vi "Ultrasonic Loop.vi"   [LabVIEW 2014]
uses:
  Common Code/Ultrasonic Indicators.ctl
  <vilib>/Rock Robotics/WPI/Ultrasonic/WPI_UltrasonicRangeUnits.ctl
  Common Code/Change Detect Boolean.vi
  <vilib>/Rock Robotics/WPI/Ultrasonic/WPI_SonarSRF04DigitalRefNum Registry Get.vi
  <vilib>/Rock Robotics/WPI/Ultrasonic/WPI_SonarSRF04DigitalGetRange.vi
  <vilib>/addons/control/pid/pid.llb/PID Control Input Filter (DBL).vi
  Robot Global Data.vi
  <vilib>/addons/control/pid/NI_PID_pid.lvlib
types:
  T1 = typedef "WPI_UltrasonicRangeUnits.ctl" = enum16{"inches", "mm"}
  T2 = typedef "Ultrasonic Indicators.ctl" = cluster{"Left Distance":dbl, "Right Distance":dbl, "Center Distance":dbl, "Left Distance Unfilter":dbl, "Right Distance Unfilter":dbl, "Center Distance Unfilter":dbl}
  T3 = typedef "WPI_UltrasonicDeviceRef.ctl" = cluster{"DevStatus":errorcluster, "Ping Digital Controller":T4, "Echo Digital Controller":T4, "Ping Channel":T5, "Echo Channel":T5, "CntIndex":T6}
  T4 = typedef "FPGA_TypedefDigitalModule.ctl" = enum16{"Controller 1"}
  T5 = typedef "FPGA_DIOChannel.ctl" = enum8{"DIO 0", "DIO 1", "DIO 2", "DIO 3", "DIO 4", "DIO 5", "DIO 6", "DIO 7", "DIO 8", "DIO 9", "DIO MXP 0", "DIO MXP 1", "DIO MXP 2", "DIO MXP 3", "DIO MXP 4", "DIO MXP 5", "DIO MXP 6", "DIO MXP 7", "DIO MXP 8", "DIO MXP 9", "DIO MXP 10", "DIO MXP 11", "DIO MXP 12", "DIO MXP 13", "DIO MXP 14", "DIO MXP 15", "Invalid"}
  T6 = typedef "FPGA_CounterCtrSystemIndex.ctl" = enum8{"Ctr 0", "Ctr 1", "Ctr 2", "Ctr 3", "Ctr 4", "Ctr 5", "Ctr 6", "Ctr 7", "Invalid"}
  T7 = typedef "WPI_AnalogChannelDevRef.ctl" = cluster{"DevStatus":errorcluster, "Controller":T8, "Analog Channel":T9}
  T8 = typedef "FPGA_TypedefAnalogModule.ctl" = enum16{"Controller 1"}
  T9 = typedef "FPGA_AIChannel.ctl" = enum8{"AI 0", "AI 1", "AI 2", "AI 3", "AI MXP 0", "AI MXP 1", "AI MXP 2", "AI MXP 3", "Invalid"}
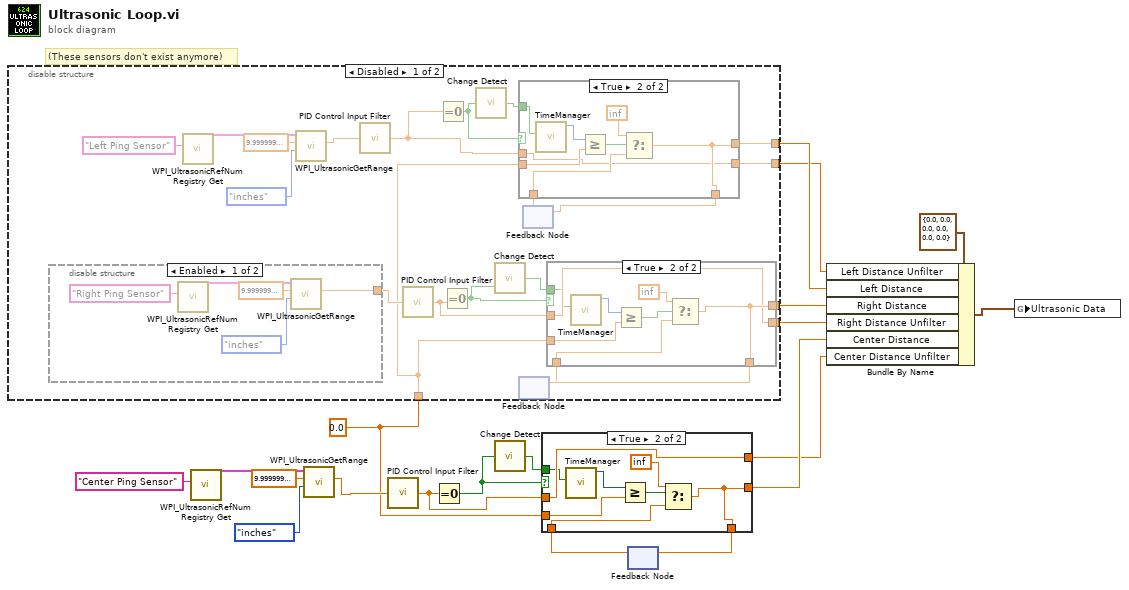
[diagram p0: block diagram]
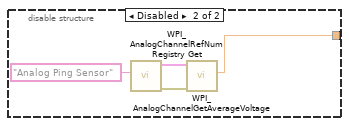
[diagram p4: hidden frame]
diagram:
  w1 = 0.0
  # "(These sensors don't exist anymore)"
  n1 = disable-structure shown="Disabled" {
    disable-tunnel: [w36 _] -> w17
    disable-tunnel: [w35 _] -> w16
    disable-tunnel: w1 -> [w26 _]
    disable-tunnel: [w25 _] -> w6
    disable-tunnel: [w24 _] -> w4
    frame Disabled {
      n2 = disable-structure shown="Enabled" {
        disable-tunnel: [w59 w64] -> w33
        frame Enabled {
          n3 = call-poly <vilib>:"WPI_UltrasonicRefNum Registry Get.vi"("refnum name"="Right Ping Sensor") -> ("SonarSRF04DevRef"=w62:T3)  [unwired: 9 in, 1 out]
          n4 = call-poly <vilib>:"WPI_UltrasonicGetRange.vi"("Range Units"=WPI_UltrasonicRangeUnits."inches", "ping time (s)"=sgl 1e-05, "SonarSRF04DevRef"=w62) -> ("Distance"=w59:dbl)  [unwired: 6 in, 2 out]
        }
        frame Disabled {
          n5 = call <vilib>:"WPI_AnalogChannelRefNum Registry Get.vi"("refnum name"="Analog Ping Sensor") -> ("error out"=w67:errorcluster, "AIDeviceRef"=w66:T7)  [unwired: 9 in]
          n6 = call <vilib>:"WPI_AnalogChannelGetAverageVoltage.vi"("error in (no error)"=w67, "AIDeviceRef"=w66) -> ("Voltage"=w64:dbl)  [unwired: 7 in, 2 out]
        }
      }
      n7 = call-poly <vilib>:"WPI_UltrasonicRefNum Registry Get.vi"("refnum name"="Left Ping Sensor") -> ("SonarSRF04DevRef"=w40:T3)  [unwired: 9 in, 1 out]
      n8 = call-poly <vilib>:"WPI_UltrasonicGetRange.vi"("Range Units"=WPI_UltrasonicRangeUnits."inches", "ping time (s)"=sgl 1e-05, "SonarSRF04DevRef"=w40) -> ("Distance"=w34:dbl)  [unwired: 6 in, 2 out]
      n9 = call-poly <vilib>:"PID Control Input Filter.vi"("input"=w34) -> ("output"=w31:dbl)  [unwired: 4 in]
      n10 = call-poly <vilib>:"PID Control Input Filter.vi"("input"=w33) -> ("output"=w32:dbl)  [unwired: 4 in]
      n11 = Equal To 0?(x=w31) -> (x = 0?=w23:bool)
      n12 = Equal To 0?(x=w32) -> (x = 0?=w21:bool)
      n13 = call-poly "Change Detect.vi"("In"=w23) -> ("Changed?"=w22:bool)
      n14 = call-poly "Change Detect.vi"("In"=w21) -> ("Changed?"=w20:bool)
      n15 = feedback #1() -> (w27:dbl)  [unwired: 1 in]
      n16 = feedback #2() -> (w29:dbl)  [unwired: 1 in]
      n17 = case shown="True" w23 {
        tunnel: [w41 w45] -> w35
        tunnel: w31 -> [w41 w43]
        tunnel: [w41 w45] -> w30
        tunnel: w29 -> [_ w46]
        tunnel: w26 -> [_ w44]
        tunnel: [w41 w43] -> w25
        tunnel: w22 -> [_ w42]
        frame False {
        }
        frame True {
          n18 = call "TimeManager.vi"("Reset?"=w42) -> ("Time Since Reset"=w49:u32)  [unwired: 9 in, 1 out]
          n19 = Greater Or Equal?(x=w49, y=w44) -> (x >= y?=w47:bool)
          n20 = Select(t=inf, s=w47, f=w46) -> (s? t:f=w45:dbl)
        }
      }
      n21 = feedback-in #2(w30) -> ()
      n22 = case shown="True" w21 {
        tunnel: [w50 w53] -> w36
        tunnel: w32 -> [w50 w52]
        tunnel: [w50 w53] -> w28
        tunnel: w27 -> [_ w55]
        tunnel: w26 -> [_ w56]
        tunnel: [w50 w52] -> w24
        tunnel: w20 -> [_ w51]
        frame False {
        }
        frame True {
          n23 = call "TimeManager.vi"("Reset?"=w51) -> ("Time Since Reset"=w57:u32)  [unwired: 9 in, 1 out]
          n24 = Greater Or Equal?(x=w57, y=w56) -> (x >= y?=w58:bool)
          n25 = Select(t=inf, s=w58, f=w55) -> (s? t:f=w53:dbl)
        }
      }
      n26 = feedback-in #1(w28) -> ()
    }
    frame Enabled {
    }
  }
  n27 = call-poly <vilib>:"WPI_UltrasonicRefNum Registry Get.vi"("refnum name"="Center Ping Sensor") -> ("SonarSRF04DevRef"=w12:T3)  [unwired: 9 in, 1 out]
  n28 = call-poly <vilib>:"WPI_UltrasonicGetRange.vi"("Range Units"=WPI_UltrasonicRangeUnits."inches", "ping time (s)"=sgl 1e-05, "SonarSRF04DevRef"=w12) -> ("Distance"=w10:dbl)  [unwired: 6 in, 2 out]
  n29 = call-poly <vilib>:"PID Control Input Filter.vi"("input"=w10) -> ("output"=w9:dbl)  [unwired: 4 in]
  n30 = Equal To 0?(x=w9) -> (x = 0?=w2:bool)
  n31 = call-poly "Change Detect.vi"("In"=w2) -> ("Changed?"=w3:bool)
  n32 = feedback #3() -> (w7:dbl)  [unwired: 1 in]
  n33 = case shown="True" w2 {
    tunnel: [w68 w71] -> w11
    tunnel: w9 -> [w68 w70]
    tunnel: [w68 w71] -> w8
    tunnel: w7 -> [_ w73]
    tunnel: w1 -> [_ w74]
    tunnel: [w68 w70] -> w5
    tunnel: w3 -> [_ w69]
    frame False {
    }
    frame True {
      n34 = call "TimeManager.vi"("Reset?"=w69) -> ("Time Since Reset"=w75:u32)  [unwired: 9 in, 1 out]
      n35 = Greater Or Equal?(x=w75, y=w74) -> (x >= y?=w76:bool)
      n36 = Select(t=inf, s=w76, f=w73) -> (s? t:f=w71:dbl)
    }
  }
  n37 = feedback-in #3(w8) -> ()
  n38 = Bundle By Name(cluster=T2 {"Left Distance"=0.0, "Right Distance"=0.0, "Center Distance"=0.0, "Left Distance Unfilter"=0.0, "Right Distance Unfilter"=0.0, "Center Distance Unfilter"=0.0} ("Ultrasonic Indicators"), "Left Distance Unfilter"=w6, "Left Distance"=w16, "Right Distance"=w17, "Right Distance Unfilter"=w4, "Center Distance"=w11, "Center Distance Unfilter"=w5) -> (w18:T2)
  n39 = global write "Robot Global Data.vi" "Ultrasonic Data"(w18) -> ()
